vi "Save Settings to XML.vi"(8 "error in (no error)":errorcluster, 11 "Settings":T1) -> (0 "error out":errorcluster)   [LabVIEW 2026, in "Settings.lvlib"]
doc: "Saves the \"User Specified\" configuration data to an XML file. This is used to remember the users settings between executions."
uses:
  Settings.lvlib
  Settings.ctl
  Acquisition/Hardware Configuration.ctl
  Logging/Logging Configuration.ctl
  <vilib>/Utility/xml.llb/Write to XML File(string).vi
  Acquisition/Acquisition.lvlib
  Logging/Logging.lvlib
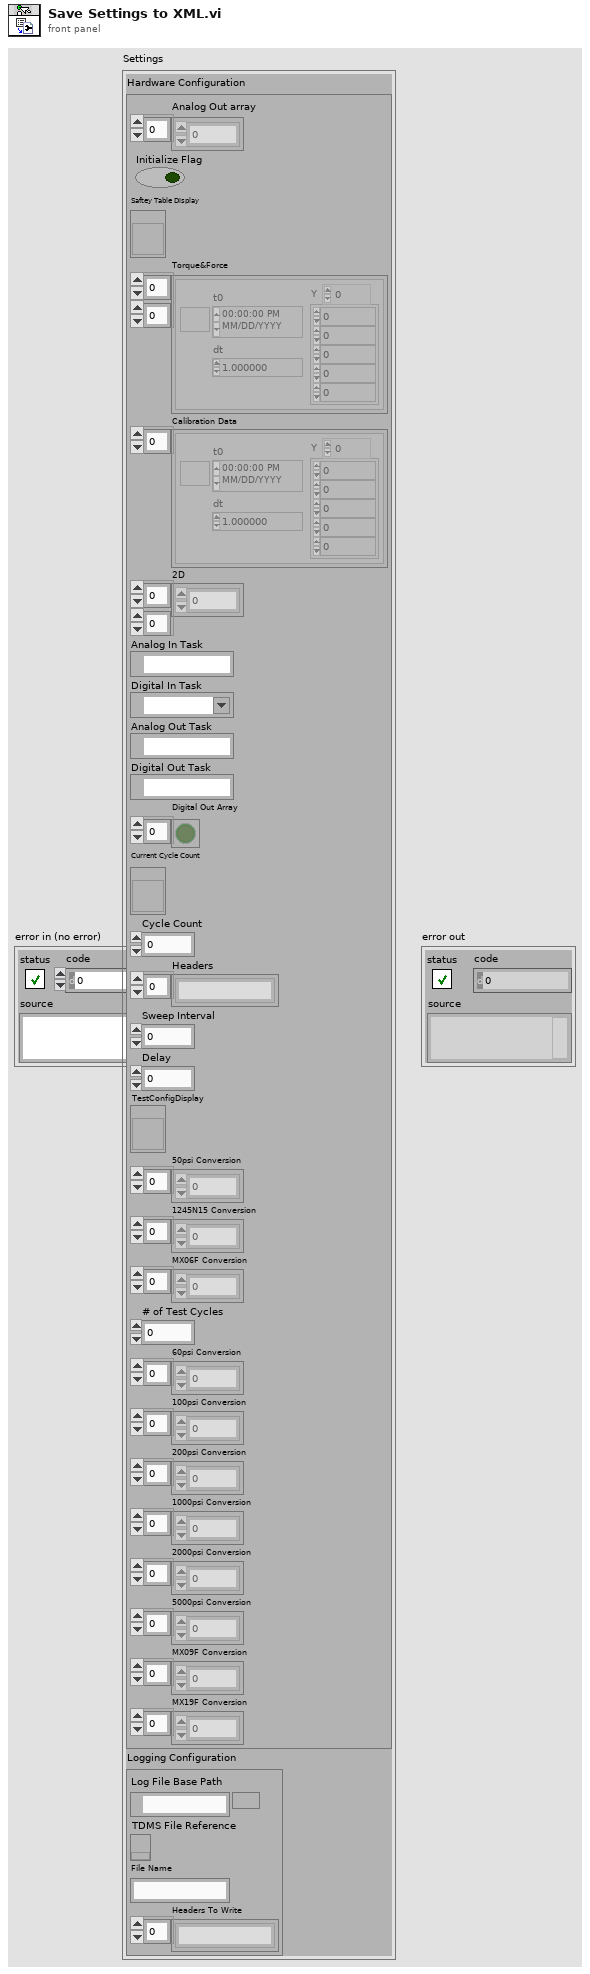
[diagram p1: front panel]
types:
  T1 = typedef "Settings.lvlib/Settings.ctl" = cluster{"Hardware Configuration":T2, "Logging Configuration":T3}
  T2 = typedef "Acquisition.lvlib/Hardware Configuration.ctl" = cluster{"Analog Out array":dbl[], "Initialize Flag":bool, "Saftey Table Display":refnum<vi>, "Torque&Force":waveform(dbl)[][], "Calibration Data":waveform(dbl)[], "2D":dbl[][], "Analog In Task":refnum<k21>, "Digital In Task":refnum<k21>, "Analog Out Task":refnum<k21>, "Digital Out Task":refnum<k21>, "Digital Out Array":bool[], "Current Cycle Count":refnum<vi>, "Cycle Count":u64, "Headers":string[], "Sweep Interval":u64, "Delay":u64, "TestConfigDisplay":refnum<vi>, "50psi Conversion":dbl[], "1245N15 Conversion":dbl[], "MX06F Conversion":dbl[], "# of Test Cycles":u64, "60psi Conversion":dbl[], "100psi Conversion":dbl[], "200psi Conversion":dbl[], "1000psi Conversion":dbl[], "2000psi Conversion":dbl[], "5000psi Conversion":dbl[], "MX09F Conversion":dbl[], "MX19F Conversion":dbl[]}
  T3 = typedef "Logging.lvlib/Logging Configuration.ctl" = cluster{"Log File Base Path":path, "TDMS File Reference":refnum<k34>, "File Name":string, "Headers To Write":string[]}
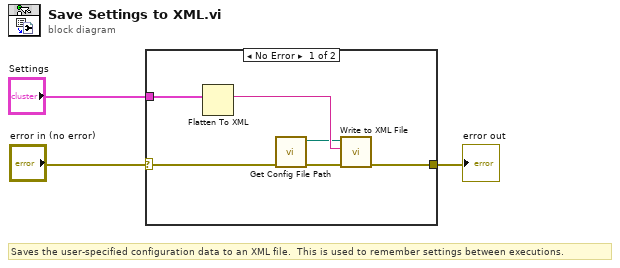
[diagram p0: block diagram]
diagram:
  # "Saves the user-specified configuration data to an XML file.  This is used to remember settings between executions."
  n1 = case shown="No Error" "error in (no error)" {
    selector: "error in (no error)" -> [w5 w10]
    tunnel: [w7 w10] -> w2
    tunnel: "Settings" -> [w9 _]
    frame No Error {
      n2 = Flatten To XML(6:w9) -> (2:w8:string)
      n3 = call "Get Config File Path.vi"("error in (no error)"=w5) -> ("error out"=w4:errorcluster, "XML File Path"=w6:path)  [unwired: 9 in]
      n4 = call-poly <vilib>:"Write to XML File.vi"("error in (no error)"=w4, "XML Input"=w8, "XML File Path"=w6) -> ("error out"=w7:errorcluster)  [unwired: 6 in, 2 out]
    }
    frame Error {
    }
  }
  "error out" <- w2
